vi "Untitled 3.vi"() -> ()   [LabVIEW 2016]
uses:
  Classes/Workspace/Workspace.ctl
  Classes/Workspace/Carrier Tray/Baseplate Tray.lvclass
  Classes/Controller/Controller.lvclass
  Classes/Workspace/Fixture.lvclass
panel:
  out "Workspace":T1
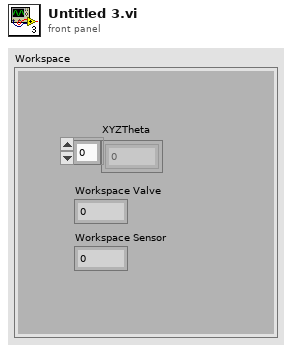
[diagram p1: front panel]
types:
  T1 = typedef "Fixture.lvclass/Workspace.ctl" = cluster{"XYZTheta":dbl[], "Workspace Valve":i32, "Workspace Sensor":i32}
  T2 = typedef "Controller.lvclass/Controllers.ctl" = cluster{"I-O.lvclass":refnum<class "I-O.lvclass">, "Motion.lvclass":refnum<class "Motion.lvclass">, "Dispenser.lvclass":refnum<class "Dispenser.lvclass">}
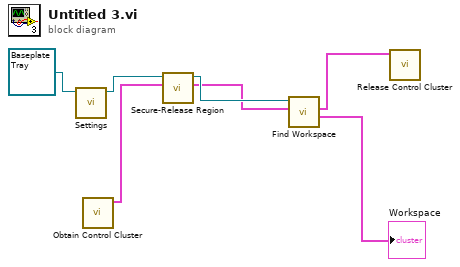
[diagram p0: block diagram]
diagram:
  n1 = call-dynamic "Settings.vi"("Baseplate Tray In"=refnum<class "Baseplate Tray.lvclass"> refnum ("Baseplate Tray.lvclass")) -> ("Baseplate Tray Out"=w4:refnum<class "Baseplate Tray.lvclass">)  [unwired: 9 in, 1 out]
  n2 = call "Obtain Control Cluster.vi"() -> ("Control Out"=w3:T2)  [unwired: 11 in]
  n3 = call-dynamic "Secure-Release Region.vi"("Control In"=w3, "Baseplate Tray in"=w4) -> ("Control Out"=w1:T2, "Baseplate Tray out"=w2:refnum<class "Baseplate Tray.lvclass">)  [unwired: 7 in, 1 out]
  n4 = call-dynamic "Find Workspace.vi"("Control In"=w1, "Baseplate Tray in"=w2) -> ("Workspace"=→"Workspace":T1, "Control Out"=w5:T2)  [unwired: 6 in, 2 out]
  n5 = call "Release Control Cluster.vi"("output cluster"=w5) -> ()  [unwired: 11 in]
